vi "Validate Handle.vi"(8 "error in":errorcluster, 10 "handle":T1 format="%02x", 11 "session in":refnum<class "Session.lvclass">) -> (0 "error out":errorcluster, 2 "valid?":bool)   [LabVIEW 2020, in "NI_SFTP.lvlib" / "Session.lvclass"]
uses:
  <vilib>/net/SFTP/Session/Session.lvclass
  <vilib>/net/SFTP/Session/Handle.ctl
  <vilib>/net/SFTP/Session/Session.lvclass/Session.ctl
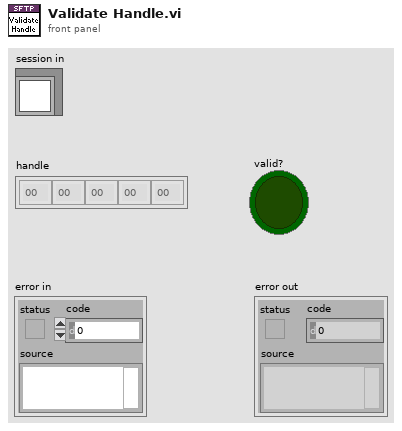
[diagram p1: front panel]
types:
  T1 = typedef "NI_SFTP.lvlib/Session.lvclass/Handle.ctl" = u8[]
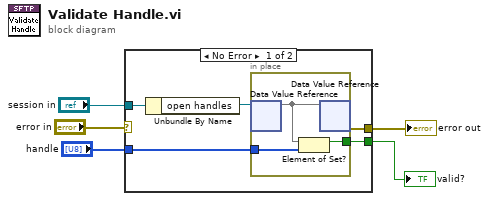
[diagram p0: block diagram]
diagram:
  n1 = case shown="No Error" "error in" {
    selector: "error in" -> [_ w14]
    tunnel: [w8 w14] -> w2
    tunnel: "session in" -> [w10 _]
    tunnel: "handle" -> [w9 _]
    tunnel: [w7 _] -> w1
    frame No Error {
      n2 = Unbundle By Name(w10) -> ("open handles"=w6:refnum<data-value>)
      n3 = in-place {
        in-place-border: w9 -> [w13]
        in-place-border: [w12] -> w7
        n4 = in-place-dvr #1(w6) -> (w11:set{T1})  [unwired: 1 out]
        n5 = Element of Set?(10:w13, 11:w11) -> (3:w12:bool)
        n6 = in-place-dvr #1(w11) -> (w8:errorcluster)  [unwired: 1 out]
      }
    }
    frame Error {
    }
  }
  "error out" <- w2
  "valid?" <- w1
